vi "adapter_rm_imu.vi"(10 "configuration_rm_imu":T1={"chunk"=4096, "mode"=1, "_reserved_0"=0, "_reserved_1"=0, "_reserved_2"=0, "_reserved_3"=0, "_reserved_4"=0, "_reserved_5"=0, "_reserved_6"=0}, 11 "path in":path=path "hl2ss_ulm.dll") -> (2 "configuration":u64, 3 "path out":path)   [LabVIEW 2023]
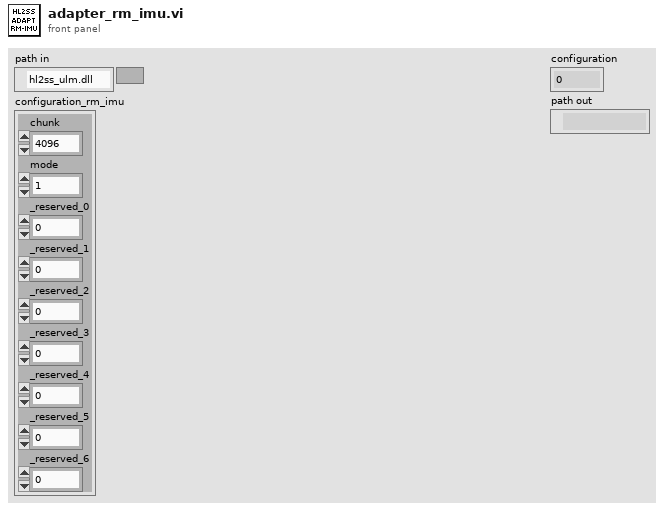
[diagram p1: front panel]
types:
  T1 = cluster{"chunk":u64, "mode":u8, "_reserved_0":u8, "_reserved_1":u8, "_reserved_2":u8, "_reserved_3":u8, "_reserved_4":u8, "_reserved_5":u8, "_reserved_6":u8}
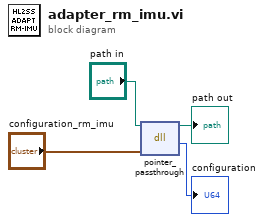
[diagram p0: block diagram]
diagram:
  n1 = dll-call lib="C:/Users/jcds/Documents/GitHub/hl2ss/extensions/client_labview/hl2ss_ulm.dll" fn="pointer_passthrough"(path in="path in", "p"="configuration_rm_imu") -> (path out=→"path out":path, "return type"=→"configuration":u64)  [unwired: 3 in, 1 out]
